vi "Connect Clock Terminals.vi"(8 "error in (no error)":errorcluster, 10 "Clock Routing":T1={"Source Terminal"="Oscillator", "Destination Terminal"="ClkOut"}, 11 "instrument handle":refnum<k15>) -> (0 "error out":errorcluster, 3 "instrument handle out":refnum<k15>)   [LabVIEW 2026]
doc: "Allow for cluster input containing clock source and destination information. Uses the NI-SYNC driver to make the connections."
uses:
  Clock Routing.ctl
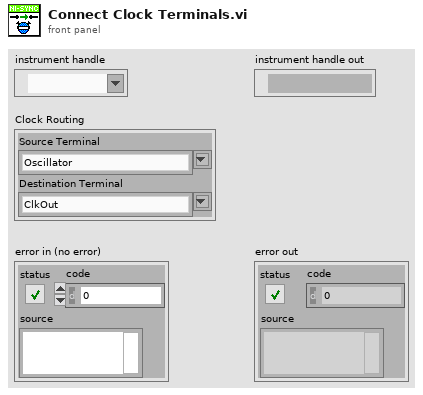
[diagram p1: front panel]
types:
  T1 = typedef "Clock Routing.ctl" = cluster{"Source Terminal":string, "Destination Terminal":string}
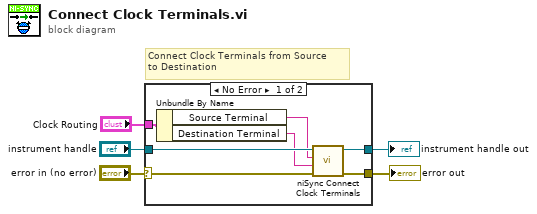
[diagram p0: block diagram]
diagram:
  # "Connect Clock Terminals from Source\nto Destination"
  n1 = case shown="No Error" "error in (no error)" {
    selector: "error in (no error)" -> [w10 w14]
    tunnel: "Clock Routing" -> [w8 _]
    tunnel: "instrument handle" -> [w12 w13]
    tunnel: [w11 w13] -> w4
    tunnel: [w9 w14] -> w2
    frame No Error {
      n2 = Unbundle By Name(w8) -> ("Source Terminal"=w7:string, "Destination Terminal"=w6:string)
      n3 = call <instrlib>:"niSync Connect Clock Terminals.vi"("error in (no error)"=w10, "destination terminal"=w6, "source terminal"=w7, "instrument handle"=w12) -> ("error out"=w9:errorcluster, "instrument handle out"=w11:refnum<k15>)  [unwired: 6 in]
    }
    frame Error {
    }
  }
  "instrument handle out" <- w4
  "error out" <- w2
